vi "InitializeECC.vi"(8 "Error In":errorcluster) -> (0 "Error Out":errorcluster)   [LabVIEW 2010]
uses:
  RScode.dll
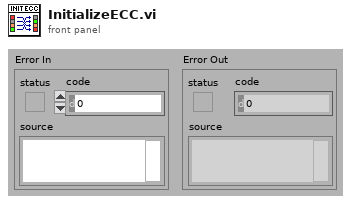
[diagram p1: front panel]
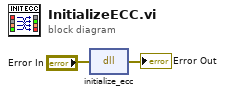
[diagram p0: block diagram]
diagram:
  n1 = dll-call lib="Z:/Ted On My Mac/GitHub/Configurator/Source/Utilities/RScode/RScode.dll" fn="initialize_ecc"(error in="Error In") -> (error out=→"Error Out":errorcluster)  [unwired: 3 in, 1 out]
